vi "Sensor Test.vi"(8 "error in (no error)":errorcluster, 11 "Test Type":string) -> (0 "Error Out":errorcluster, 2 "Error String":string, 3 "Passed?":bool)   [LabVIEW 2014]
uses:
  CAN Communication/PAS/PAS.lvclass
  CAN Communication/PAS/Typedefs/Pressure Sensor.ctl
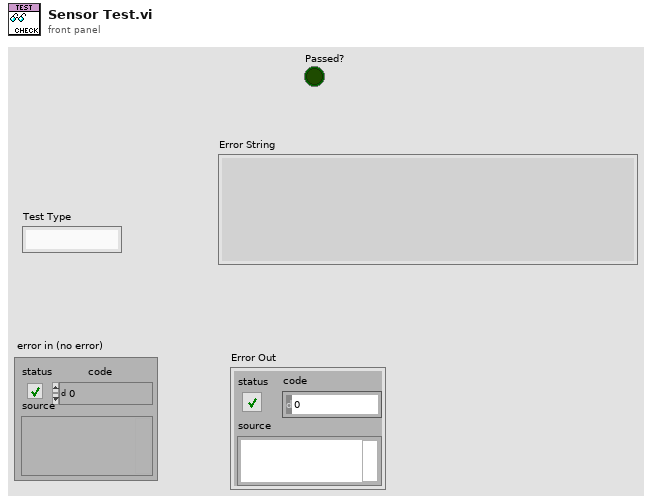
[diagram p1: front panel]
types:
  T1 = typedef "PAS.lvclass/Pressure Sensor.ctl" = u16
  T2 = typedef "PAS.lvclass/Session Handle.ctl" = refnum<data-value>
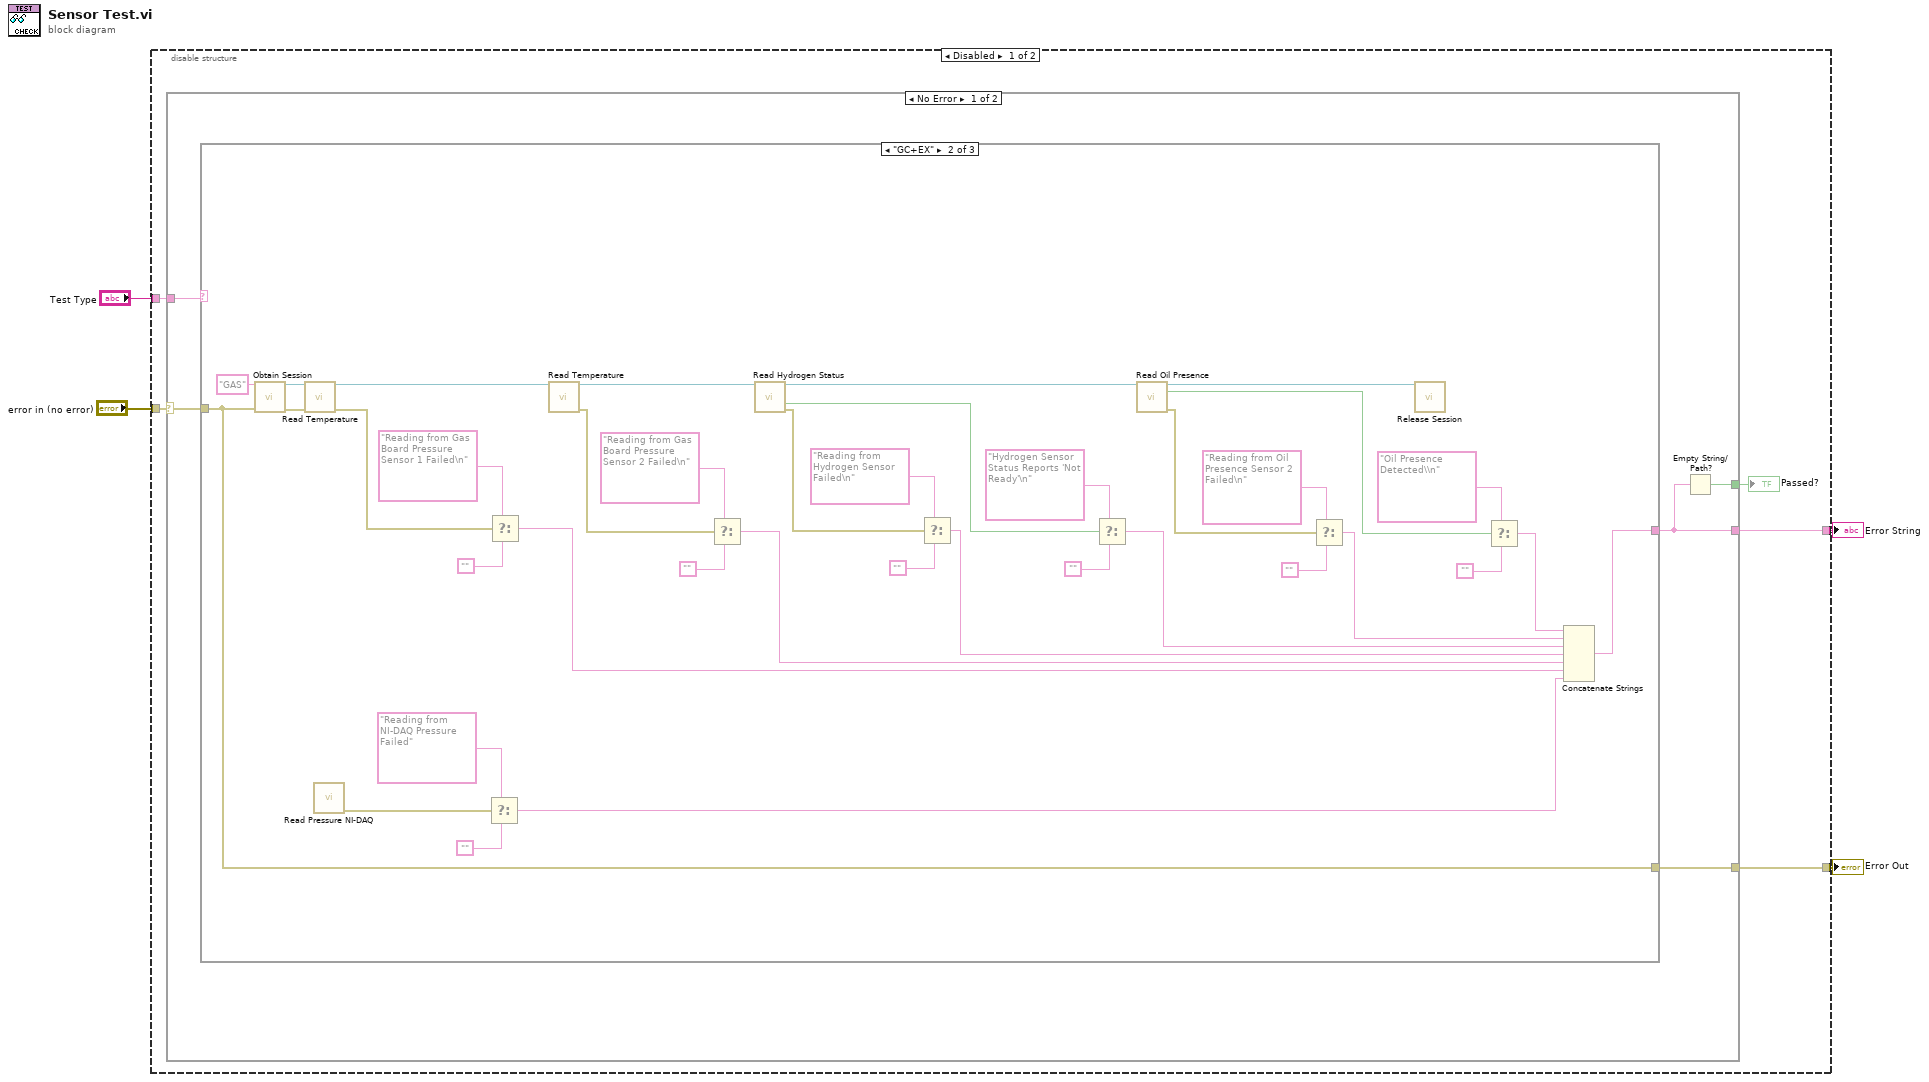
[diagram p0: block diagram]
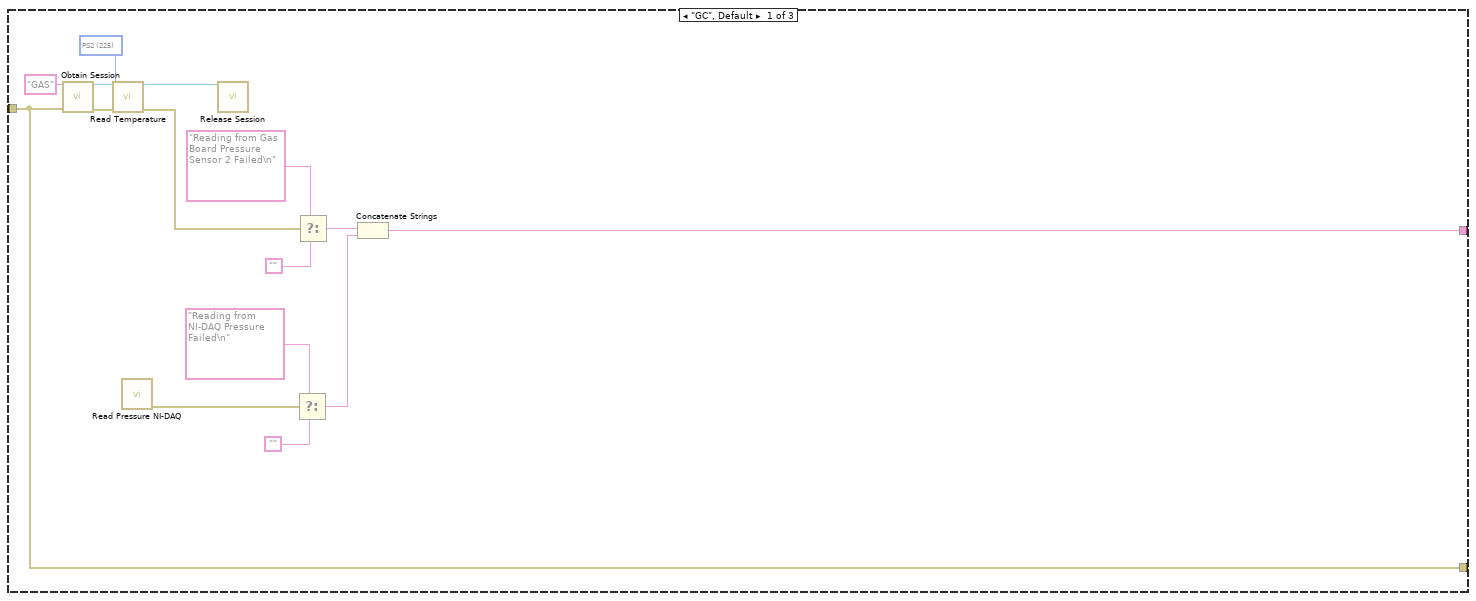
[diagram p2: hidden frame]
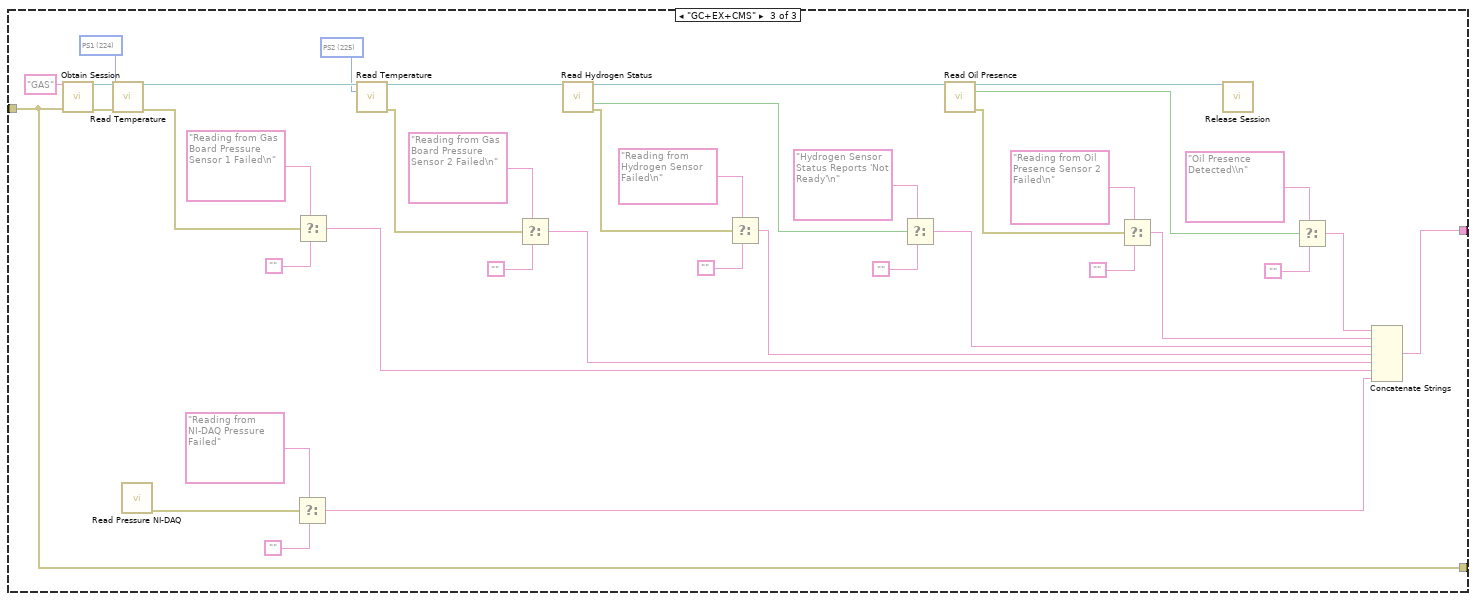
[diagram p3: hidden frame]
diagram:
  n1 = disable-structure shown="Disabled" {
    disable-tunnel: "Test Type" -> [w9 _]
    disable-tunnel: "error in (no error)" -> [w8 _]
    disable-tunnel: [w7 _] -> w2
    disable-tunnel: [w6 _] -> w1
    frame Disabled {
      n2 = case shown="No Error" w8 {
        selector: w8 -> [w13 w106]
        tunnel: w9 -> [w14 _]
        tunnel: [w11 _] -> w7
        tunnel: [w12 w106] -> w6
        tunnel: [w10 _] -> w5
        frame No Error {
          n3 = case shown="\"GC+EX\"" w14 {
            tunnel: w13 -> [w15 w30 w67]
            tunnel: [w16 w31 w68] -> w11
            tunnel: [w15 w30 w67] -> w12
            frame "GC", Default {
              w28 = T1 225 items=["PS1"=224, "PS2"=225] ("Pressure Sensor")
              n4 = call "Obtain Session.vi"("Session  Name ()"="GAS", "error in (no error)"=w15) -> ("Session Handle"=w27:T2, "error out"=w25:errorcluster)  [unwired: 12 in]
              n5 = call "Read Temperature.vi"("Session Handle in"=w27, 5:w28, "error in (no error)"=w25) -> ("Session Handle out"=w26:T2, "error out"=w24:errorcluster)  [unwired: 10 in, 1 out]
              n6 = call "Read Pressure NI-DAQ.vi"() -> ("error out"=w18:errorcluster)  [unwired: 10 in, 1 out]
              n7 = call "Release Session.vi"("Session Handle"=w26) -> ()  [unwired: 14 in, 1 out]
              n8 = Select(t="Reading from NI-DAQ Pressure Failed\n", s=w18, f="") -> (s? t:f=w17:string)
              n9 = Select(t="Reading from Gas Board Pressure Sensor 2 Failed\n", s=w24, f="") -> (s? t:f=w21:string)
              n10 = Concatenate Strings(w21, w17) -> (w16:string)
            }
            frame "GC+EX" {
              n11 = call "Obtain Session.vi"("Session  Name ()"="GAS", "error in (no error)"=w30) -> ("Session Handle"=w65:T2, "error out"=w64:errorcluster)  [unwired: 12 in]
              n12 = call "Read Temperature.vi"("Session Handle in"=w65, "error in (no error)"=w64) -> ("Session Handle out"=w55:T2, "error out"=w63:errorcluster)  [unwired: 11 in, 1 out]
              n13 = call "Read Pressure NI-DAQ.vi"() -> ("error out"=w58:errorcluster)  [unwired: 10 in, 1 out]
              n14 = Select(t="Reading from NI-DAQ Pressure Failed", s=w58, f="") -> (s? t:f=w32:string)
              n15 = Select(t="Reading from Gas Board Pressure Sensor 1 Failed\n", s=w63, f="") -> (s? t:f=w33:string)
              n16 = call "Read Temperature.vi"("Session Handle in"=w55) -> ("Session Handle out"=w53:T2, "error out"=w54:errorcluster)  [unwired: 12 in, 1 out]
              n17 = Select(t="Reading from Gas Board Pressure Sensor 2 Failed\n", s=w54, f="") -> (s? t:f=w34:string)
              n18 = call "Read Hydrogen Status.vi"("Session Handle in"=w53) -> ("Ready?"=w47:bool, "Session Handle out"=w46:T2, "error out"=w50:errorcluster)  [unwired: 9 in, 3 out]
              n19 = Select(t="Reading from Hydrogen Sensor Failed\n", s=w50, f="") -> (s? t:f=w35:string)
              n20 = Select(t="Hydrogen Sensor Status Reports 'Not Ready'\n", s=w47, f="") -> (s? t:f=w36:string)
              n21 = call "Read Oil Presence.vi"("Session Handle in"=w46) -> ("Session Handle out"=w39:T2, "Present?"=w40:bool, "error out"=w41:errorcluster)  [unwired: 12 in]
              n22 = Select(t="Reading from Oil Presence Sensor 2 Failed\n", s=w41, f="") -> (s? t:f=w37:string)
              n23 = call "Release Session.vi"("Session Handle"=w39) -> ()  [unwired: 14 in, 1 out]
              n24 = Select(t="Oil Presence Detected\\n", s=w40, f="") -> (s? t:f=w38:string)
              n25 = Concatenate Strings(w38, w37, w36, w35, w34, w33, w32) -> (w31:string)
            }
            frame "GC+EX+CMS" {
              w92 = T1 225 items=["PS1"=224, "PS2"=225] ("Pressure Sensor")
              w104 = T1 224 items=["PS1"=224, "PS2"=225] ("Pressure Sensor")
              n26 = call "Obtain Session.vi"("Session  Name ()"="GAS", "error in (no error)"=w67) -> ("Session Handle"=w103:T2, "error out"=w102:errorcluster)  [unwired: 12 in]
              n27 = call "Read Temperature.vi"("Session Handle in"=w103, 5:w104, "error in (no error)"=w102) -> ("Session Handle out"=w93:T2, "error out"=w101:errorcluster)  [unwired: 10 in, 1 out]
              n28 = call "Read Pressure NI-DAQ.vi"() -> ("error out"=w96:errorcluster)  [unwired: 10 in, 1 out]
              n29 = Select(t="Reading from NI-DAQ Pressure Failed", s=w96, f="") -> (s? t:f=w69:string)
              n30 = Select(t="Reading from Gas Board Pressure Sensor 1 Failed\n", s=w101, f="") -> (s? t:f=w70:string)
              n31 = call "Read Temperature.vi"("Session Handle in"=w93, 5:w92) -> ("Session Handle out"=w90:T2, "error out"=w91:errorcluster)  [unwired: 11 in, 1 out]
              n32 = Select(t="Reading from Gas Board Pressure Sensor 2 Failed\n", s=w91, f="") -> (s? t:f=w71:string)
              n33 = call "Read Hydrogen Status.vi"("Session Handle in"=w90) -> ("Ready?"=w84:bool, "Session Handle out"=w83:T2, "error out"=w87:errorcluster)  [unwired: 9 in, 3 out]
              n34 = Select(t="Reading from Hydrogen Sensor Failed\n", s=w87, f="") -> (s? t:f=w72:string)
              n35 = Select(t="Hydrogen Sensor Status Reports 'Not Ready'\n", s=w84, f="") -> (s? t:f=w73:string)
              n36 = call "Read Oil Presence.vi"("Session Handle in"=w83) -> ("Session Handle out"=w76:T2, "Present?"=w77:bool, "error out"=w78:errorcluster)  [unwired: 12 in]
              n37 = Select(t="Reading from Oil Presence Sensor 2 Failed\n", s=w78, f="") -> (s? t:f=w74:string)
              n38 = call "Release Session.vi"("Session Handle"=w76) -> ()  [unwired: 14 in, 1 out]
              n39 = Select(t="Oil Presence Detected\\n", s=w77, f="") -> (s? t:f=w75:string)
              n40 = Concatenate Strings(w75, w74, w73, w72, w71, w70, w69) -> (w68:string)
            }
          }
          n41 = Empty String/Path?(string/path=w11) -> (empty?=w10:bool)
        }
        frame Error {
        }
      }
      "Passed?" <- w5
    }
    frame Enabled {
    }
  }
  "Error String" <- w2
  "Error Out" <- w1
